vi "dfd_Dummy_FIRTEngine.vi"(0 "input data":fxp<+/-,64,32>, 1 "Output_Latch":bool, 5 "Input_Latch":bool=TRUE, 7 "coefficients":fxp<+/-,16,1>[](array[numeric])=[0.0] format="%.16g", 11 "opState":T1) -> (4 "output data":fxp<+/-,64,32>)   [LabVIEW 2017]
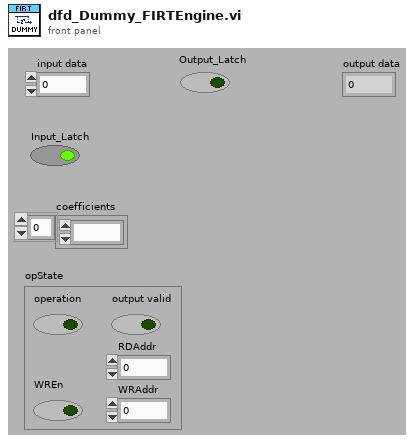
[diagram p1: front panel]
types:
  T1 = cluster{"operation":bool, "RDAddr":u16, "WREn":bool, "WRAddr":u16, "output valid":bool}
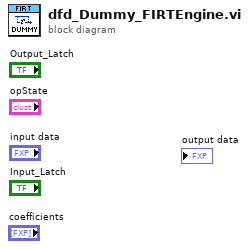
[diagram p0: block diagram]
diagram:
